vi "Set Instruments.vi"(8 "error in (no error)":errorcluster, 10 "Instrument info":T1={"instrumentPid"="Undocumented", "title"="", "filename"="", "filestorePath"="", "createDate"="Undocumented activity", "modifyDate"="", "categories"="", "instrumenType"=""}, 11 "Log Record in":refnum<class "Log Record.lvclass">) -> (0 "error out":errorcluster, 3 "Log Record out":refnum<class "Log Record.lvclass">)   [LabVIEW 2024, in "Log Record.lvclass"]
uses:
  Log Record.lvclass
  Log Record.lvclass/Log Record.ctl
  NHMFL_Core/Libraries/FAIR Data/MagX/Instrument info.ctl
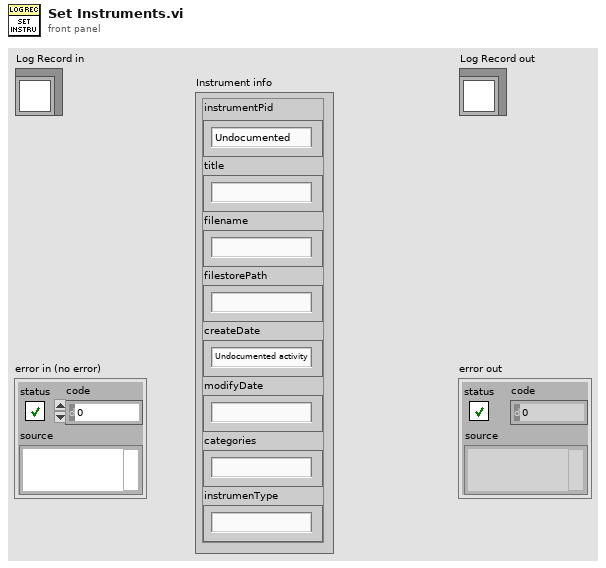
[diagram p1: front panel]
types:
  T1 = typedef "Instrument info.ctl" = cluster{"instrumentPid":string, "title":string, "filename":string, "filestorePath":string, "createDate":string, "modifyDate":string, "categories":string, "instrumenType":string}
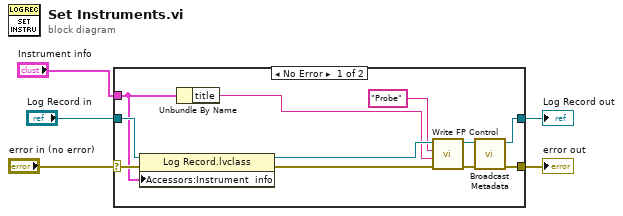
[diagram p0: block diagram]
diagram:
  n1 = case shown="No Error" "error in (no error)" {
    selector: "error in (no error)" -> [w16 w18]
    tunnel: [w8 w18] -> w4
    tunnel: [w9 w17] -> w2
    tunnel: "Log Record in" -> [w15 w17]
    tunnel: "Instrument info" -> [w12 _]
    frame No Error {
      n2 = property class="Log Record.lvclass"(reference=w15, error in=w16, "Accessors:Instrument  info"=w12) -> (reference out=w14:refnum<class "Log Record.lvclass">, error out=w7:errorcluster)
      n3 = Unbundle By Name(w12) -> ("title"=w11:string)
      n4 = call-dynamic "Write FP Control.vi"("error in (no error)"=w7, "Control Value"=w11, "Control Name"="Probe", "Measure Object in"=w14) -> ("error out"=w6:errorcluster, "Measure Object out"=w10:refnum<class "Log Record.lvclass">)  [unwired: 6 in]
      n5 = call-dynamic "Broadcast Metadata.vi"("error in (no error)"=w6, "Log Record in"=w10) -> ("error out"=w8:errorcluster, "Log Record out"=w9:refnum<class "Log Record.lvclass">)  [unwired: 8 in]
    }
    frame Error {
    }
  }
  "error out" <- w4
  "Log Record out" <- w2
